vi "Globals.vi"() -> ()   [LabVIEW 2019]
panel:
  in  "min neighbors":i32
  in  "max width":i32
  in  "min width":i32
  in  "scale factor":dbl
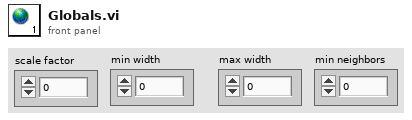
[diagram p1: front panel]
diagram:
